vi "ep_Read Public Event Inf.vi"(8 "error in (no error)":errorcluster, 11 "task in":T2={"file refnums"=[], "Data Object"=refnum, "config info"={"station_name"="", "rec_dev_id"="", "rev_year"=1999.0, "TT"=0, "##A"=0, "##D"=0, "analog channel info"=[], "status channel info"=[], "lf"=50.0, "nrates"=0, "samp info"=[], "initial timestamp"=timestamp(0 s since 1904-01-01), "trigger timestamp"=timestamp(0 s since 1904-01-01), "ft"=enum."Binary", "timemult"=1.0}, "public inf content"={"Source"="", "Record Type"=enum."Unknown", "Phase ID"="", "Event Description"="", "Device ID"="", "Distance of Fault"=-1.0, "Distance Unit"=enum."Miles", "Max_Current"=inf, "Min_Current"=-inf, "Max_Voltage"=inf, "Min_Voltage"=-inf, "EventNoteCount"=0, "Event Information"=[]}, "private inf content"=[], "internal buffers"={"start index"=1, "config to public inf"=enum."disabled", "static config info"="", "static file_des record inf"="", "static file_des channel inf"="", "public inf"="", "private inf"=""}} {"public inf content"."Event Information"."min sample number" max=9999999999; "public inf content"."Event Information"."max sample number" max=9999999999; "config info"."nrates" max=999; "config info"."status channel info"."Dn" min=1 max=999999; "config info"."analog channel info"."An" min=1 max=999999; "config info"."trigger timestamp" format="%<%H:%M:%S%6u\n%d/%m/%Y>T"; "config info"."initial timestamp" format="%<%H:%M:%S%6u\n%d/%m/%Y>T"; "config info"."##D" max=999999; "config info"."##A" max=999999; "config info"."TT" min=1 max=999999; "config info"."rev_year" min=1999.0 max=1999.0}) -> (0 "error out":errorcluster, 2 "public event information":T1[](array[typedef]) {"min sample number" max=9999999999; "max sample number" max=9999999999}, 3 "task out":T2={"file refnums"=[], "Data Object"=refnum, "config info"={"station_name"="", "rec_dev_id"="", "rev_year"=1999.0, "TT"=0, "##A"=0, "##D"=0, "analog channel info"=[], "status channel info"=[], "lf"=50.0, "nrates"=0, "samp info"=[], "initial timestamp"=timestamp(0 s since 1904-01-01), "trigger timestamp"=timestamp(0 s since 1904-01-01), "ft"=enum."Binary", "timemult"=1.0}, "public inf content"={"Source"="", "Record Type"=enum."Unknown", "Phase ID"="", "Event Description"="", "Device ID"="", "Distance of Fault"=-1.0, "Distance Unit"=enum."Miles", "Max_Current"=inf, "Min_Current"=-inf, "Max_Voltage"=inf, "Min_Voltage"=-inf, "EventNoteCount"=0, "Event Information"=[]}, "private inf content"=[], "internal buffers"={"start index"=1, "config to public inf"=enum."disabled", "static config info"="", "static file_des record inf"="", "static file_des channel inf"="", "public inf"="", "private inf"=""}} {"public inf content"."Event Information"."min sample number" max=9999999999; "public inf content"."Event Information"."max sample number" max=9999999999; "config info"."nrates" max=999; "config info"."status channel info"."Dn" min=1 max=999999; "config info"."analog channel info"."An" min=1 max=999999; "config info"."trigger timestamp" format="%<%H:%M:%S%6u\n%d/%m/%Y>T"; "config info"."initial timestamp" format="%<%H:%M:%S%6u\n%d/%m/%Y>T"; "config info"."##D" max=999999; "config info"."##A" max=999999; "config info"."TT" min=1 max=999999; "config info"."rev_year" min=1999.0 max=1999.0})   [LabVIEW 2011, in "NI_EP_COMTRADE.lvlib"]
uses:
  <vilib>/addons/Electrical Power/File IO/NI_EP_COMTRADE.lvlib
  <vilib>/addons/Electrical Power/File IO/COMTRADE/typedefs/ep_Task.ctl
  <vilib>/addons/Electrical Power/File IO/COMTRADE/typedefs/ep_Config Info.ctl
  <vilib>/addons/Electrical Power/File IO/COMTRADE/typedefs/ep_Analog Channel Info.ctl
  <vilib>/addons/Electrical Power/File IO/COMTRADE/typedefs/ep_Status Channel Info.ctl
  <vilib>/addons/Electrical Power/File IO/COMTRADE/typedefs/ep_File Format.ctl
  <vilib>/addons/Electrical Power/File IO/COMTRADE/typedefs/ep_Public Inf Content.ctl
  <vilib>/addons/Electrical Power/File IO/COMTRADE/typedefs/ep_Public Event Inf.ctl
  <vilib>/addons/Electrical Power/File IO/COMTRADE/typedefs/ep_Private Inf Content.ctl
  <vilib>/Platform/storage/Storage.llb/Get Property (Storage Refnums).vi
  <vilib>/Platform/storage/Storage.llb/Get Property (I32).vi
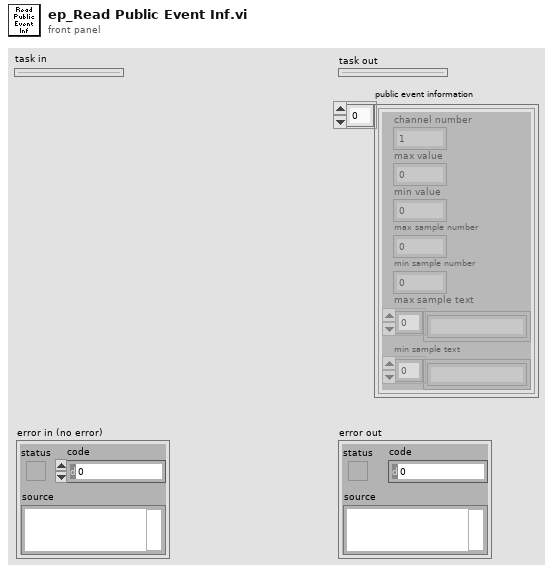
[diagram p1: front panel]
types:
  T1 = typedef "NI_EP_COMTRADE.lvlib/ep_Public Event Inf.ctl" = cluster{"channel number":u32, "max value":dbl, "min value":dbl, "max sample number":u64, "min sample number":u64, "max sample text":string[], "min sample text":string[]}
  T2 = typedef "NI_EP_COMTRADE.lvlib/ep_Task.ctl" = cluster{"file refnums":refnum<file>[], "Data Object":refnum<k20>, "config info":T3, "public inf content":T7, "private inf content":T8, "internal buffers":cluster{"start index":u32, "config to public inf":enum16{"disabled", "enabled", "buffered"}, "static config info":string, "static file_des record inf":string, "static file_des channel inf":string, "public inf":string, "private inf":string}}
  T3 = typedef "NI_EP_COMTRADE.lvlib/ep_Config Info.ctl" = cluster{"station_name":string, "rec_dev_id":string, "rev_year":dbl, "TT":u32, "##A":u32, "##D":u32, "analog channel info":T4[], "status channel info":T5[], "lf":sgl, "nrates":u16, "samp info":cluster{"samp":sgl, "endsamp":u32}[], "initial timestamp":timestamp, "trigger timestamp":timestamp, "ft":T6, "timemult":sgl}
  T4 = typedef "NI_EP_COMTRADE.lvlib/ep_Analog Channel Info.ctl" = cluster{"An":u32, "ch_id":string, "ph":string, "ccbm":string, "uu":string, "a":sgl, "b":sgl, "skew":sgl, "min":i32, "max":i32, "primary":sgl, "secondary":sgl, "PS":enum16{"P", "S"}}
  T5 = typedef "NI_EP_COMTRADE.lvlib/ep_Status Channel Info.ctl" = cluster{"Dn":u32, "ch_id":string, "ph":string, "ccbm":string, "Y":bool}
  T6 = typedef "NI_EP_COMTRADE.lvlib/ep_File Format.ctl" = enum16{"ASCII", "Binary"}
  T7 = typedef "NI_EP_COMTRADE.lvlib/ep_Public Inf Content.ctl" = cluster{"Source":string, "Record Type":enum16{"Fault", "Unknown", "Misoperation", "Close", "Trip", "Reclose", "Power swing", "Simulation"}, "Phase ID":string, "Event Description":string, "Device ID":string, "Distance of Fault":dbl, "Distance Unit":enum16{"Miles", "Kilometers", "Percent of line", "Percent of setting", "Ohms"}, "Max_Current":dbl, "Min_Current":dbl, "Max_Voltage":dbl, "Min_Voltage":dbl, "EventNoteCount":u32, "Event Information":T1[]}
  T8 = typedef "NI_EP_COMTRADE.lvlib/ep_Private Inf Content.ctl" = cluster{"Section Header":string, "Entry Names":string[], "Entry Values":string[]}[]
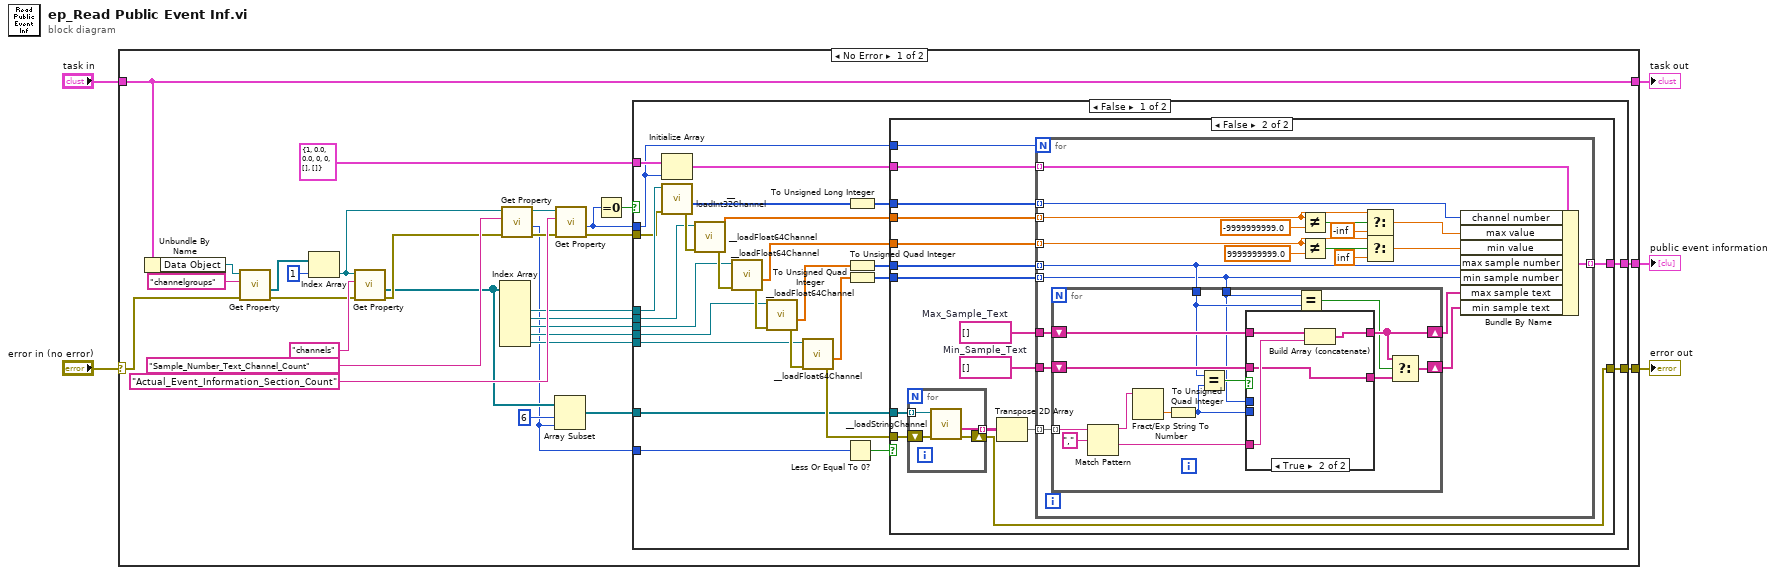
[diagram p0: block diagram]
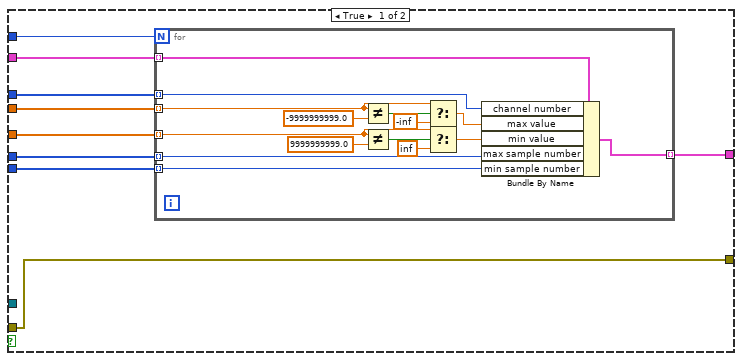
[diagram p2: hidden frame]
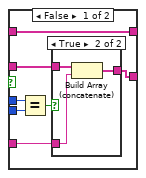
[diagram p3: hidden frame]
diagram:
  n1 = case shown="No Error" "error in (no error)" {
    selector: "error in (no error)" -> [w29 w156]
    tunnel: "task in" -> [w34 w157]
    tunnel: [w34 w157] -> w3
    tunnel: [w25 w156] -> w2
    tunnel: [w26 _] -> w1
    frame No Error {
      n2 = Unbundle By Name(w34) -> ("Data Object"=w33:refnum<k20>)
      n3 = call-poly <vilib>:"Get Property.vi"("error in (no error)"=w29, "Property name"="channelgroups", "storage refnum"=w33) -> ("error out"=w6:errorcluster, "Value"=w32:refnum<k20>[])  [unwired: 6 in, 1 out]
      n4 = Index Array(array=w32, index=1) -> (element=w21:refnum<k20>)
      n5 = call-poly <vilib>:"Get Property.vi"("error in (no error)"=w6, "Property name"="channels", "storage refnum"=w21) -> ("error out"=w22:errorcluster, "Value"=w20:refnum<k20>[])  [unwired: 6 in, 1 out]
      n6 = Index Array(array=w20) -> (element #2=w14:refnum<k20>, element #3=w15:refnum<k20>, element #4=w17:refnum<k20>, element #5=w16:refnum<k20>, element #6=w18:refnum<k20>)  [unwired: 6 in, 1 out]
      n7 = call-poly <vilib>:"Get Property.vi"("error in (no error)"=w22, "Property name"="Sample_Number_Text_Channel_Count", "storage refnum"=w21) -> ("error out"=w13:errorcluster, "Value"=w7:i32, "storage refnum out"=w12:refnum<k20>)  [unwired: 6 in]
      n8 = Array Subset(array=w20, index=6, length=w7) -> (w10:refnum<k20>[])
      n9 = call-poly <vilib>:"Get Property.vi"("error in (no error)"=w13, "Property name"="Actual_Event_Information_Section_Count", "storage refnum"=w12) -> ("error out"=w11:errorcluster, "Value"=w9:i32)  [unwired: 6 in, 1 out]
      n10 = Equal To 0?(x=w9) -> (x = 0?=w8:bool)
      n11 = case shown="False" w8 {
        tunnel: T1 {"channel number"=1, "max value"=0.0, "min value"=0.0, "max sample number"=0, "min sample number"=0, "max sample text"=[], "min sample text"=[]} ("Cluster") -> [w61 _]
        tunnel: [w46 _] -> w26
        tunnel: [w45 w155] -> w25
        tunnel: w9 -> [w44 _]
        tunnel: w18 -> [w43 _]
        tunnel: w17 -> [w42 _]
        tunnel: w16 -> [w41 _]
        tunnel: w15 -> [w40 _]
        tunnel: w14 -> [w39 _]
        tunnel: w11 -> [w38 w155]
        tunnel: w10 -> [w37 _]
        tunnel: w7 -> [w36 _]
        frame False {
          n12 = Initialize Array(w61, w44) -> (w60:T1[])
          n13 = call <vilib>:"__loadInt32Channel.vi"("error in (no error)"=w38, "Data object in"=w39) -> ("error out"=w59:errorcluster, "Values"=w53:i32[])  [unwired: 2 in, 2 out]
          n14 = call <vilib>:"__loadFloat64Channel.vi"("error in (no error)"=w59, "Data object in"=w40) -> ("error out"=w58:errorcluster, "Values"=w55:dbl[])  [unwired: 2 in, 2 out]
          n15 = call <vilib>:"__loadFloat64Channel.vi"("error in (no error)"=w58, "Data object in"=w42) -> ("error out"=w57:errorcluster, "Values"=w54:dbl[])  [unwired: 2 in, 2 out]
          n16 = call <vilib>:"__loadFloat64Channel.vi"("error in (no error)"=w57, "Data object in"=w41) -> ("error out"=w56:errorcluster, "Values"=w50:dbl[])  [unwired: 2 in, 2 out]
          n17 = call <vilib>:"__loadFloat64Channel.vi"("error in (no error)"=w56, "Data object in"=w43) -> ("error out"=w47:errorcluster, "Values"=w49:dbl[])  [unwired: 2 in, 2 out]
          n18 = Less Or Equal To 0?(x=w36) -> (x <= 0?=w35:bool)
          n19 = To Unsigned Long Integer(number=w53) -> (unsigned 32bit integer=w52:u32[])
          n20 = To Unsigned Quad Integer(1:w50) -> (0:w51:u64[])
          n21 = To Unsigned Quad Integer(1:w49) -> (0:w48:u64[])
          n22 = case shown="False" w35 {
            tunnel: w60 -> [w70 w100]
            tunnel: w55 -> [w69 w99]
            tunnel: w54 -> [w68 w98]
            tunnel: w52 -> [w67 w96]
            tunnel: w51 -> [w66 w95]
            tunnel: w48 -> [w65 w94]
            tunnel: w47 -> [w62 w93]
            tunnel: [w64 w89] -> w46
            tunnel: [w62 w88] -> w45
            tunnel: w44 -> [w63 w87]
            tunnel: w37 -> [_ w86]
            frame True {
              n23 = for {
                N: w63 -> [_]
                tunnel: w70 -> [w85] mode=indexing
                tunnel: w67 -> [w84] mode=indexing
                tunnel: w69 -> [w75] mode=indexing
                tunnel: w68 -> [w81] mode=indexing
                tunnel: w66 -> [w72] mode=indexing
                tunnel: w65 -> [w71] mode=indexing
                tunnel: [w83] -> w64 mode=indexing
                n24 = Not Equal?(x=w75, y=-9999999999.0 ("f")) -> (x != y?=w77:bool)
                n25 = Not Equal?(x=w81, y=9999999999.0 ("f")) -> (x != y?=w79:bool)
                n26 = Select(t=w75, s=w77, f=-inf) -> (s? t:f=w76:dbl)
                n27 = Select(t=w81, s=w79, f=inf) -> (s? t:f=w82:dbl)
                n28 = Bundle By Name(cluster=w85, "channel number"=w84, "max value"=w76, "min value"=w82, "max sample number"=w72, "min sample number"=w71) -> (w83:T1)
              }
            }
            frame False {
              w90 = string[] []  # Min_Sample_Text
              w91 = string[] []  # Max_Sample_Text
              n29 = for {
                tunnel: w86 -> [w104] mode=indexing
                tunnel: [w103] -> w97 mode=indexing
                shift-right: [w101] -> w88
                shift-left: w93 -> [w102]
                n30 = call <vilib>:"__loadStringChannel.vi"("error in (no error)"=w102, "Data object in"=w104) -> ("error out"=w101:errorcluster, "Values"=w103:string[])  [unwired: 2 in, 2 out]
              }
              n31 = Transpose 2D Array(2D array=w97) -> (transposed array=w92:string[][])
              n32 = for {
                N: w87 -> [_]
                tunnel: w100 -> [w124] mode=indexing
                tunnel: w96 -> [w123] mode=indexing
                tunnel: w99 -> [w109] mode=indexing
                tunnel: w98 -> [w115] mode=indexing
                tunnel: w95 -> [w106] mode=indexing
                tunnel: w94 -> [w105] mode=indexing
                tunnel: w92 -> [w122] mode=indexing
                tunnel: w91 -> [w121]
                tunnel: w90 -> [w120]
                tunnel: [w117] -> w89 mode=indexing
                n33 = for {
                  tunnel: w122 -> [w137] mode=indexing
                  tunnel: w106 -> [w127]
                  shift-right: [w129] -> w119
                  shift-left: w121 -> [w139]
                  tunnel: w105 -> [w126]
                  shift-right: [w130] -> w118
                  shift-left: w120 -> [w138]
                  n34 = Match Pattern(string=w137, regular expression="," ("search string/char (-)")) -> (before substring=w135:string, after substring=w134:string)  [unwired: 1 in, 2 out]
                  n35 = Fract/Exp String To Number(string=w135) -> (number=w133:dbl)  [unwired: 3 in, 1 out]
                  n36 = To Unsigned Quad Integer(1:w133) -> (0:w132:u64)
                  n37 = Equal?(x=w127, y=w132) -> (x = y?=w131:bool)
                  n38 = case shown="True" w131 {
                    tunnel: w139 -> [w144 w154]
                    tunnel: w134 -> [w145 w153]
                    tunnel: [w144 w152] -> w129
                    tunnel: w126 -> [w142 _]
                    tunnel: w138 -> [w146 w151]
                    tunnel: [w143 w151] -> w128
                    tunnel: w132 -> [w141 _]
                    frame False {
                      n39 = Equal?(x=w142, y=w141) -> (x = y?=w140:bool)
                      n40 = case shown="True" w140 {
                        tunnel: w146 -> [w147 w150]
                        tunnel: w145 -> [_ w149]
                        tunnel: [w147 w148] -> w143
                        frame False {
                        }
                        frame True {
                          n41 = Build Array (concatenate)(w150, w149) -> (w148:string[])
                        }
                      }
                    }
                    frame True {
                      n42 = Build Array (concatenate)(w154, w153) -> (w152:string[])
                    }
                  }
                  n43 = Equal?(x=w126, y=w127) -> (x = y?=w125:bool)
                  n44 = Select(t=w129, s=w125, f=w128) -> (s? t:f=w130:string[])
                }
                n45 = Not Equal?(x=w109, y=-9999999999.0 ("f")) -> (x != y?=w111:bool)
                n46 = Not Equal?(x=w115, y=9999999999.0 ("f")) -> (x != y?=w113:bool)
                n47 = Select(t=w109, s=w111, f=-inf) -> (s? t:f=w110:dbl)
                n48 = Select(t=w115, s=w113, f=inf) -> (s? t:f=w116:dbl)
                n49 = Bundle By Name(cluster=w124, "channel number"=w123, "max value"=w110, "min value"=w116, "max sample number"=w106, "min sample number"=w105, "max sample text"=w119, "min sample text"=w118) -> (w117:T1)
              }
            }
          }
        }
        frame True {
        }
      }
    }
    frame Error {
    }
  }
  "task out" <- w3
  "error out" <- w2
  "public event information" <- w1
